vi "controlBusWhatNext.vi"(11 "busIn":T1) -> (2 "whereNext":T2, 3 "busOut":T1)   [LabVIEW 2016]
uses:
  AalborgServerStates.ctl
  AalborgServerControlBus.ctl
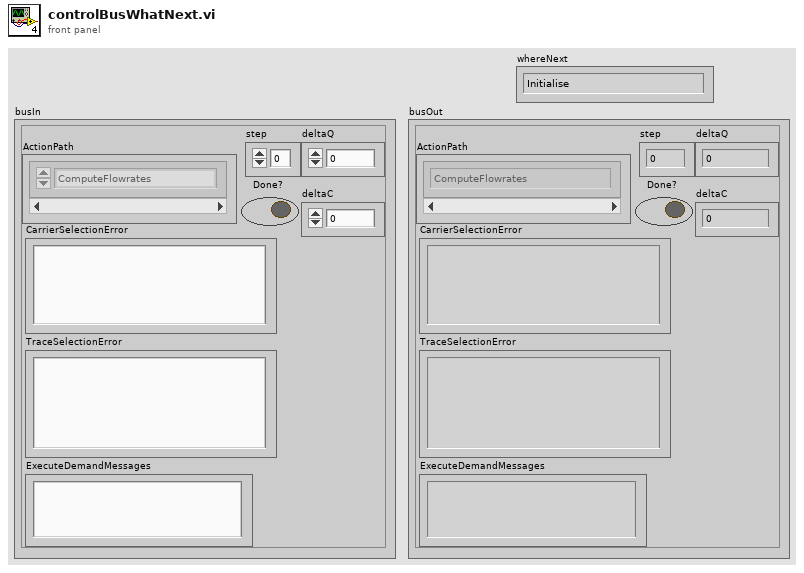
[diagram p1: front panel]
types:
  T1 = typedef "AalborgServerControlBus.ctl" = cluster{"ActionPath":T2[], "step":i32, "Done?":bool, "CarrierSelectionError":string, "TraceSelectionError":string, "ExecuteDemandMessages":string, "deltaQ":dbl, "deltaC":dbl}
  T2 = typedef "AalborgServerStates.ctl" = enum16{"Initialise", "Supervise", "WhatNext", "ComputeFlowrates", "ADAMiseDemands", "ListMFCchannels", "ChooseMFCs", "CalculateSetpoints", "ExecuteSetpoints", "CloseAll", "Summarise"}
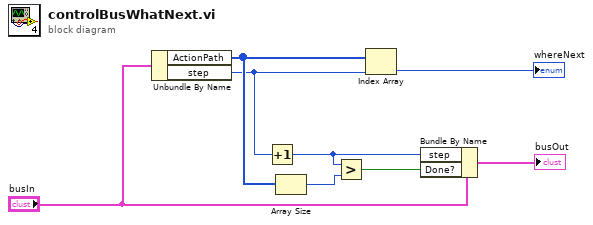
[diagram p0: block diagram]
diagram:
  n1 = Unbundle By Name("busIn") -> ("ActionPath"=w5:T2[], "step"=w2:i32)
  n2 = Increment(x=w2) -> (x+1=w1:i32)
  n3 = Array Size(array=w5) -> (size(s)=w4:i32)
  n4 = Greater?(x=w1, y=w4) -> (0:w3:bool)
  n5 = Index Array(array=w5, index=w2) -> (element=→"whereNext":T2)
  n6 = Bundle By Name(cluster="busIn", "step"=w1, "Done?"=w3) -> (→"busOut":T1)
